vi "Mars3D_old.vi"(7 "Statemachine Data IN":T2={"Impulse Positions"=[], "Old Impulse positions for Undo"=[], "No. Imp"=0, "Parameter Time Series"=[], "Parameter Impuls Series"=[], "Experiment Parameters"={"Freq"=0.0, "Vel"=0, "Acc"=0, "Stimulus"=""}, "Autosort File"=refnum, "Data File"={"Data Channels"=[], "Sample Rate"=0, "Channel List"=[]}, "Experiment data path"=path "/Macintosh HD/Users/patrick/Studium/Diploma Thesis/Data Analysis", "Image data path"=path "/Macintosh HD/Users/patrick/Studium/Diploma Thesis/Data Analysis", "LVS data path"=path "/Macintosh HD/Users/patrick/Studium/Diploma Thesis/Data Analysis", "Raw copy path"=path "/Macintosh HD/Users/patrick/Studium/Diploma Thesis/Data Analysis", "filename"="No file selected", "desaccading parameters"={"Tolerance"=0, "Acc Range"=0.0, "Sample Rate"=0, "Impulse Plane 2"=enum."Other", "Impulse dir"=FALSE}, "Experiment Parameters 2"={"Subject"="", "Strain"="", "Rotation plane"="", "Experimenter"="", "Trial"=0.0, "Time"=0.0}, "Excel"={"Excel._Application"=refnum, "Use Excel"=FALSE, "Worksheet SINE"=refnum, "Row SINE"=0, "Worksheet TRANS"=refnum, "Row TRANS"=0}, "Session Config File"=refnum, "Autosort Parameter Set"=1, "EMA Version"="", "desacc "={"Threshold 1 [Acc]"=1617.080808080808, "Threshold 2 [% of TH1]"=67, "tolerance"=5, "Search WD "=0.19090909090909092, " always use TH2"=TRUE, "Range"=3.2323232323232323, "Max time"=200.0, "Min time"=20.0, "Velocity Threshold"=67}, "Cycle Nr for Saccades"={"POS"=0, "NEG"=0}, "Undo Counter"=0, "History Length"=0, "Redo Counter"=0, "Histpry Position"=0, "Raw Data File"={"Data Channels"=[], "Sample Rate"=0, "Channel List"=[]}, "calibration name"="No file selected"} {"Parameter Time Series"."time offset" format="%.3f"; "Parameter Time Series"."Gain" format="%.1f"; "Parameter Time Series"."Offset" format="%.1f"; "Parameter Time Series"."List 1" items=["Motor-Pos", "Motor-Vel", "Lx Position-in-Head", "Ly Position-in-Head", "Lz Position-in-Head", "Lx Velocity-in-Head", "Ly Velocity-in-Head", "Lz Velocity-in-Head", "Ll Velocity-in-Head", "Lr Velocity-in-Head", "Lx Accel-in-Head", "Ly Accel-in-Head", "Lz Accel-in-Head", "Rx Position-in-Head", "Ry Position-in-Head", "Rz Position-in-Head", "Rx Velocity-in-Head", "Ry Velocity-in-Head", "Rz Velocity-in-Head", "Rl Velocity-in-Head", "Rr Velocity-in-Head", "Rx Accel-in-Head", "Ry Accel-in-Head", "Rz Accel-in-Head", "Global Trigger", "", "", ""]; "Parameter Impuls Series"."Gain" format="%.1f"; "Parameter Impuls Series"."Offset" format="%.1f"}) -> (1 "stop 3":bool, 3 "Data Output":T1={"Data Channels"=array24x25400[609600 elements], "Sample Rate"=200, "Channel List"=["Chair Position", "Chair Velocity", "Lx Position-in-Head", "Ly Position-in-Head", "Lz Position-in-Head", "Lx Velocity-in-Head", "Ly Velocity-in-Head", "Lz Velocity-in-Head", "Ll Velocity-in-Head", "Lr Velocity-in-Head", "Lx Accel-in-Head", "Ly Accel-in-Head", "Lz Accel-in-Head", "Rx Position-in-Head", "Ry Position-in-Head", "Rz Position-in-Head", "Rx Velocity-in-Head", "Ry Velocity-in-Head", "Rz Velocity-in-Head", "Rl Velocity-in-Head", "Rr Velocity-in-Head", "Rx Accel-in-Head", "Ry Accel-in-Head", "Rz Accel-in-Head"]} {"Data Channels" format="%.2f"}, 5 "Statemachine Data OUT":T2={"Impulse Positions"=[], "Old Impulse positions for Undo"=[], "No. Imp"=0, "Parameter Time Series"=[], "Parameter Impuls Series"=[], "Experiment Parameters"={"Freq"=0.0, "Vel"=0, "Acc"=0, "Stimulus"=""}, "Autosort File"=refnum, "Data File"={"Data Channels"=[], "Sample Rate"=0, "Channel List"=[]}, "Experiment data path"=path "/Macintosh HD/Users/patrick/Studium/Diploma Thesis/Data Analysis", "Image data path"=path "/Macintosh HD/Users/patrick/Studium/Diploma Thesis/Data Analysis", "LVS data path"=path "/Macintosh HD/Users/patrick/Studium/Diploma Thesis/Data Analysis", "Raw copy path"=path "/Macintosh HD/Users/patrick/Studium/Diploma Thesis/Data Analysis", "filename"="No file selected", "desaccading parameters"={"Tolerance"=0, "Acc Range"=0.0, "Sample Rate"=0, "Impulse Plane 2"=enum."Other", "Impulse dir"=FALSE}, "Experiment Parameters 2"={"Subject"="", "Strain"="", "Rotation plane"="", "Experimenter"="", "Trial"=0.0, "Time"=0.0}, "Excel"={"Excel._Application"=refnum, "Use Excel"=FALSE, "Worksheet SINE"=refnum, "Row SINE"=0, "Worksheet TRANS"=refnum, "Row TRANS"=0}, "Session Config File"=refnum, "Autosort Parameter Set"=1, "EMA Version"="", "desacc "={"Threshold 1 [Acc]"=1617.080808080808, "Threshold 2 [% of TH1]"=67, "tolerance"=5, "Search WD "=0.19090909090909092, " always use TH2"=TRUE, "Range"=3.2323232323232323, "Max time"=200.0, "Min time"=20.0, "Velocity Threshold"=67}, "Cycle Nr for Saccades"={"POS"=0, "NEG"=0}, "Undo Counter"=0, "History Length"=0, "Redo Counter"=0, "Histpry Position"=0, "Raw Data File"={"Data Channels"=[], "Sample Rate"=0, "Channel List"=[]}, "calibration name"="No file selected"} {"Parameter Time Series"."time offset" format="%.3f"; "Parameter Time Series"."Gain" format="%.1f"; "Parameter Time Series"."Offset" format="%.1f"; "Parameter Time Series"."List 1" items=["Motor-Pos", "Motor-Vel", "Lx Position-in-Head", "Ly Position-in-Head", "Lz Position-in-Head", "Lx Velocity-in-Head", "Ly Velocity-in-Head", "Lz Velocity-in-Head", "Ll Velocity-in-Head", "Lr Velocity-in-Head", "Lx Accel-in-Head", "Ly Accel-in-Head", "Lz Accel-in-Head", "Rx Position-in-Head", "Ry Position-in-Head", "Rz Position-in-Head", "Rx Velocity-in-Head", "Ry Velocity-in-Head", "Rz Velocity-in-Head", "Rl Velocity-in-Head", "Rr Velocity-in-Head", "Rx Accel-in-Head", "Ry Accel-in-Head", "Rz Accel-in-Head", "Global Trigger", "", "", ""]; "Parameter Impuls Series"."Gain" format="%.1f"; "Parameter Impuls Series"."Offset" format="%.1f"})   [LabVIEW 2016]
uses:
  core/type-defs/TD_Statemachine-Data.ctl
  core/type-defs/TD_Time Series.ctl
  core/type-defs/TD_Impulse Parameter.ctl
  <vilib>/Utility/file.llb/Read From Spreadsheet File (DBL).vi
  tracking algorithmus/3 dot tracker.lvlib
  core/core.lvlib
panel:
  in  "stop 2":bool
  in  "VOG system":enum16{"Mouse", "Chinchilla"}(ring)
  in  "Tab Control":T5(tab)
  in  "Right Eye":T6 {"y" format="%.2f"; "z" format="%.2f"; "theta" format="%.2f"; "phi" format="%.2f"; "d" format="%.2f"}
  in  "Left Eye":T6 {"y" format="%.2f"; "z" format="%.2f"; "theta" format="%.2f"; "phi" format="%.2f"; "d" format="%.2f"}
  in  "Position Convention":u16(ring)=1 items=["Fick Angles", "Rotation Vectors"]
  in  "Angles":bool
  in  "Time Stamp":timestamp
  in  "Savgol":bool
  in  "Plot Selection":T3 {"time offset" format="%.3f"; "Gain" format="%.1f"; "Offset" format="%.1f"; "List 1" items=["Motor-Pos", "Motor-Vel", "Lx Position-in-Head", "Ly Position-in-Head", "Lz Position-in-Head", "Lx Velocity-in-Head", "Ly Velocity-in-Head", "Lz Velocity-in-Head", "Ll Velocity-in-Head", "Lr Velocity-in-Head", "Lx Accel-in-Head", "Ly Accel-in-Head", "Lz Accel-in-Head", "Rx Position-in-Head", "Ry Position-in-Head", "Rz Position-in-Head", "Rx Velocity-in-Head", "Ry Velocity-in-Head", "Rz Velocity-in-Head", "Rl Velocity-in-Head", "Rr Velocity-in-Head", "Rx Accel-in-Head", "Ry Accel-in-Head", "Rz Accel-in-Head", "Global Trigger", "", "", ""]}
  in  "Plot Selection 2":T4=[{"Color"=4652800, "Visible"=TRUE, "Channel"=1, "Invert"=FALSE, "Desaccade"=FALSE, "Offset"=0.0, "Gain"=1.0}, {"Color"=16860, "Visible"=TRUE, "Channel"=7, "Invert"=FALSE, "Desaccade"=FALSE, "Offset"=0.0, "Gain"=1.0}, {"Color"=16711680, "Visible"=TRUE, "Channel"=18, "Invert"=FALSE, "Desaccade"=FALSE, "Offset"=0.0, "Gain"=1.0}] {"Gain" format="%.1f"; "Offset" format="%.1f"}
  in  "Tolerance":i32(slide)=40 step=2 scale=0.0..100.0
  in  "Acc Range":dbl(slide)=3000.0 step=50.0 scale=0.0..30000.0
  in  "Impulse dir":bool
  in  "Impulse Plane 2":T7(ring)=enum."Yaw" caption="Impulse Plane"
  in  "process":bool
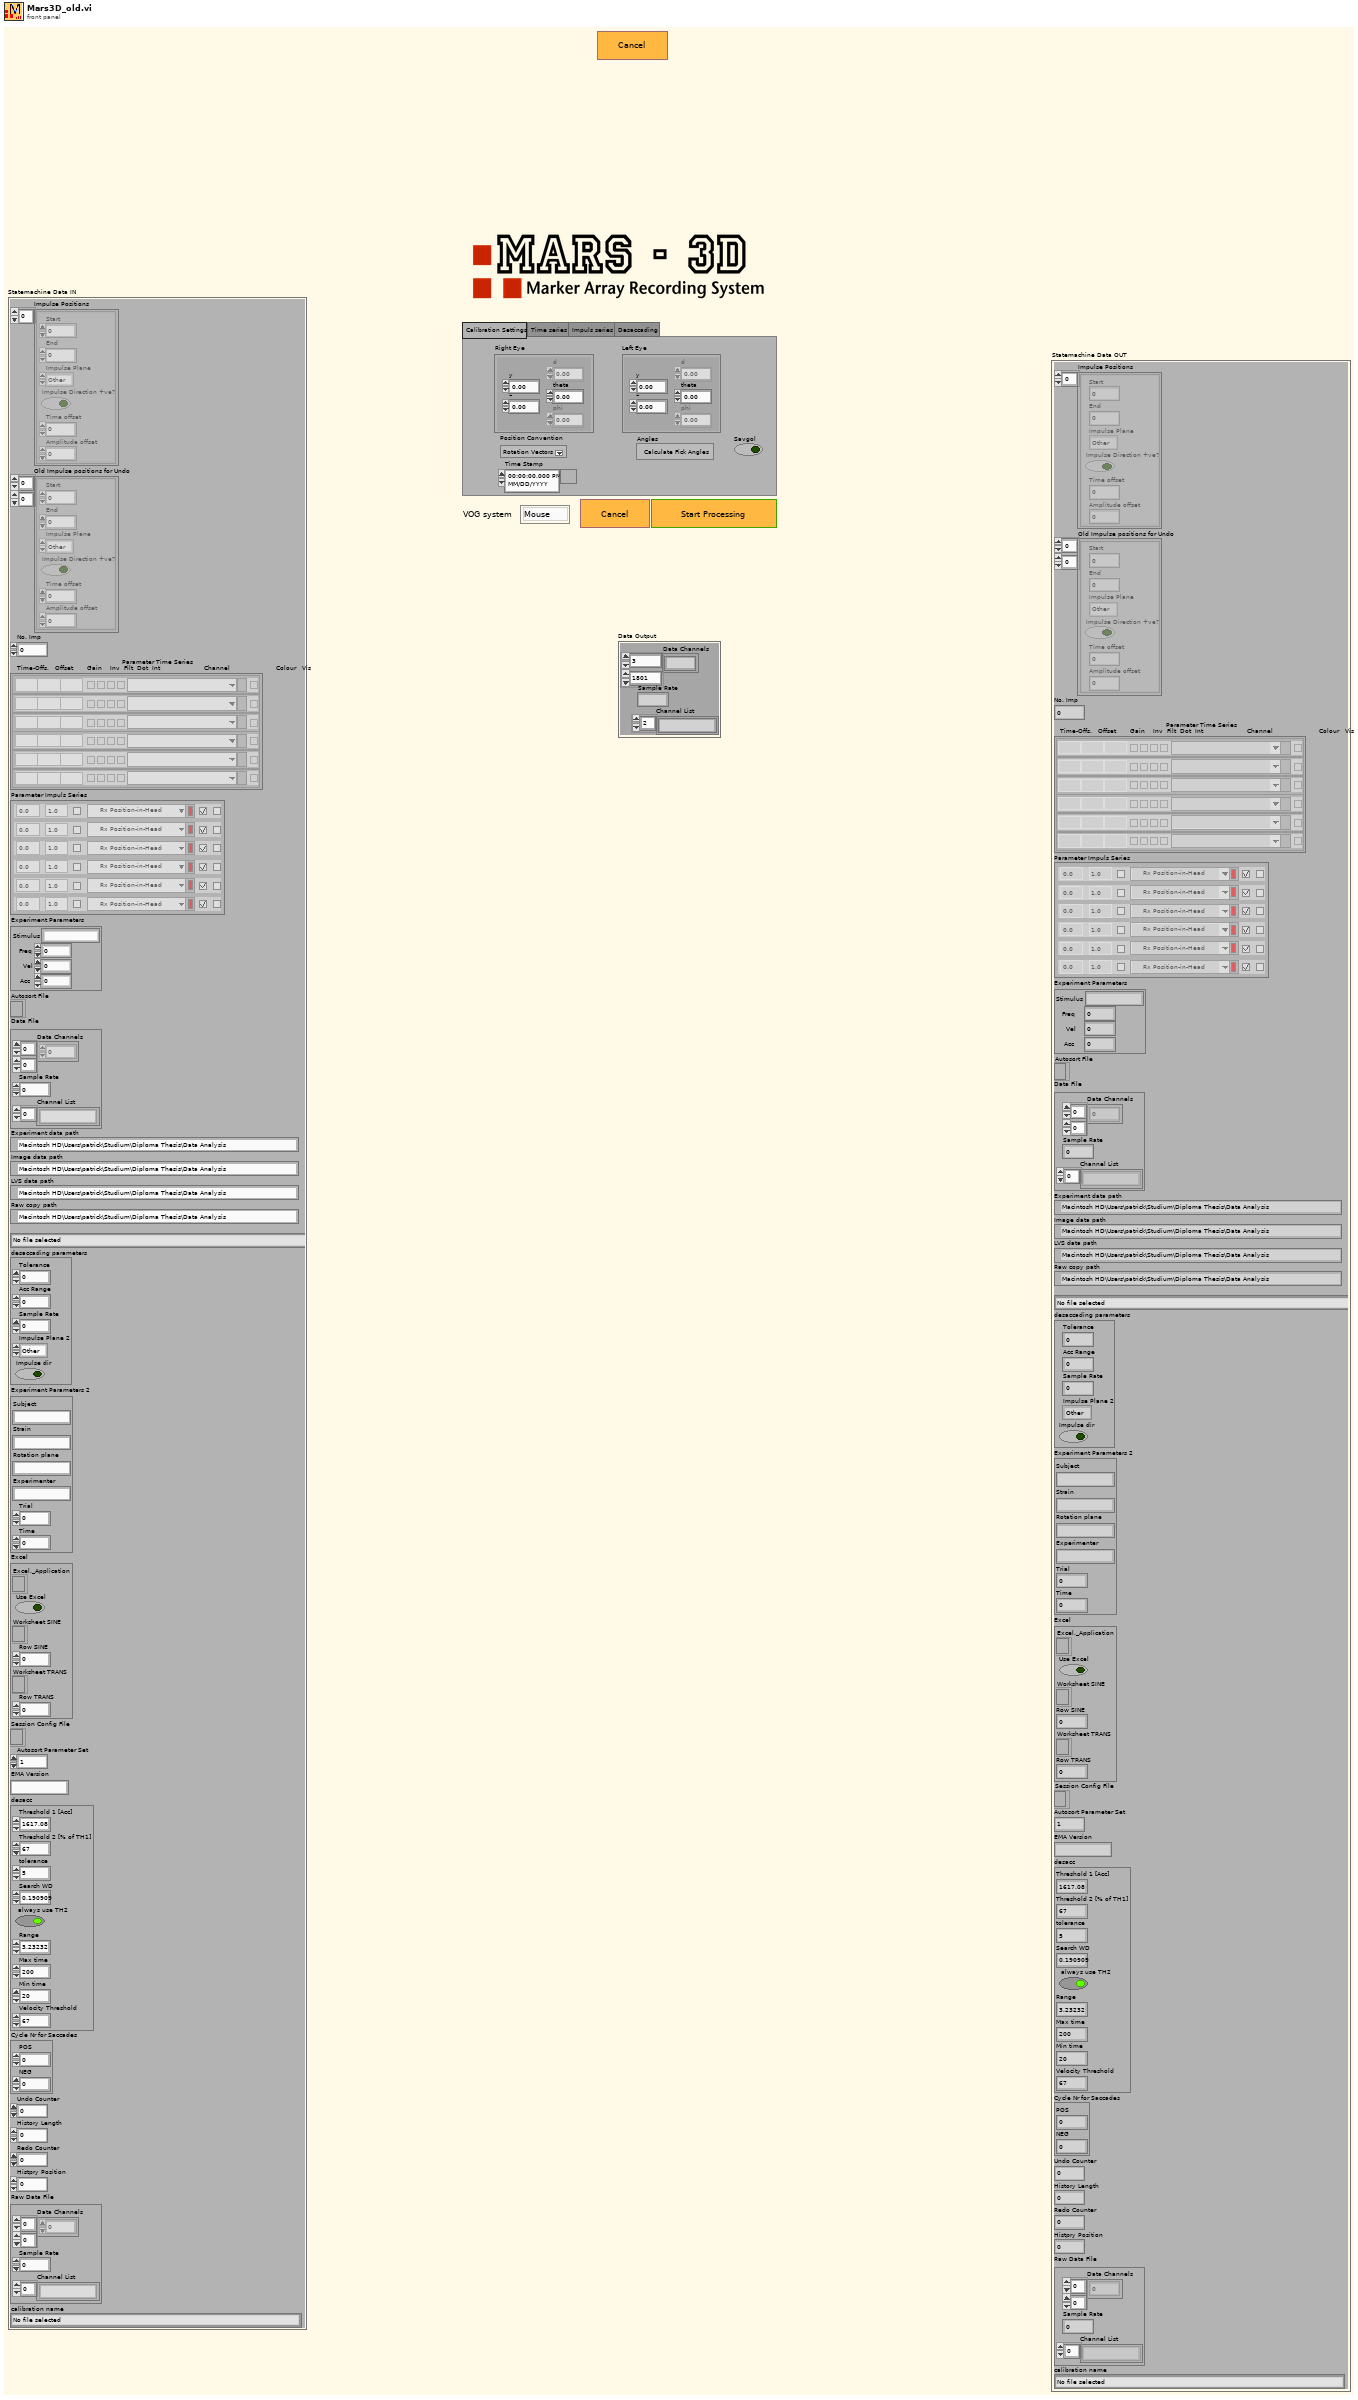
[diagram p1: front panel]
types:
  T1 = cluster{"Data Channels":dbl[][], "Sample Rate":i32, "Channel List":string[]}
  T2 = typedef "core.lvlib/TD_Statemachine-Data.ctl" = cluster{"Impulse Positions":cluster{"Start":i32, "End":i32, "Impulse Plane":enum16{"Other", "Yaw", "Pitch", "Roll", "LARP", "RALP"}, "Impulse Direction +ve?":bool, "Time offset":i32, "Amplitude offset":dbl}[], "Old Impulse positions for Undo":cluster{"Start":i32, "End":i32, "Impulse Plane":enum16{"Other", "Yaw", "Pitch", "Roll", "LARP", "RALP"}, "Impulse Direction +ve?":bool, "Time offset":i32, "Amplitude offset":dbl}[][], "No. Imp":i32, "Parameter Time Series":T3, "Parameter Impuls Series":T4, "Experiment Parameters":cluster{"Freq":dbl, "Vel":i32, "Acc":i32, "Stimulus":string}, "Autosort File":refnum<file>, "Data File":cluster{"Data Channels":dbl[][], "Sample Rate":i32, "Channel List":string[]}, "Experiment data path":path, "Image data path":path, "LVS data path":path, "Raw copy path":path, "filename":string, "desaccading parameters":cluster{"Tolerance":i32, "Acc Range":dbl, "Sample Rate":i32, "Impulse Plane 2":enum16{"Other", "Yaw", "Pitch", "Roll", "LARP", "RALP"}, "Impulse dir":bool}, "Experiment Parameters 2":cluster{"Subject":string, "Strain":string, "Rotation plane":string, "Experimenter":string, "Trial":dbl, "Time":dbl}, "Excel":cluster{"Excel._Application":refnum<k7>, "Use Excel":bool, "Worksheet SINE":refnum<k7>, "Row SINE":i32, "Worksheet TRANS":refnum<k7>, "Row TRANS":i32}, "Session Config File":refnum<file>, "Autosort Parameter Set":i32, "EMA Version":string, "desacc ":cluster{"Threshold 1 [Acc]":dbl, "Threshold 2 [% of TH1]":i32, "tolerance":i32, "Search WD ":dbl, " always use TH2":bool, "Range":dbl, "Max time":dbl, "Min time":dbl, "Velocity Threshold":i32}, "Cycle Nr for Saccades":cluster{"POS":i32, "NEG":i32}, "Undo Counter":i32, "History Length":i32, "Redo Counter":i32, "Histpry Position":i32, "Raw Data File":cluster{"Data Channels":dbl[][], "Sample Rate":i32, "Channel List":string[]}, "calibration name":string}
  T3 = typedef "core.lvlib/TD_Time Series.ctl" = cluster{"time offset":dbl, "Offset":dbl, "Gain":dbl, "inverse":bool, "filter data":bool, "dots":bool, "interpolate":bool, "List 1":u16, "Color Box":u32, "Boolean":bool}[]
  T4 = typedef "core.lvlib/TD_Impulse Parameter.ctl" = cluster{"Color":u32, "Visible":bool, "Channel":u16, "Invert":bool, "Desaccade":bool, "Offset":dbl, "Gain":dbl}[]
  T5 = enum32{"Calibration Settings", "Time series", "Impuls series", "Desaccading"}
  T6 = cluster{"d":dbl, "phi":dbl, "theta":dbl, "z":dbl, "y":dbl}
  T7 = enum16{"Other", "Yaw", "Pitch", "Roll", "LARP", "RALP"}
  T8 = cluster{"Tolerance":i32, "Acc Range":dbl, "Sample Rate":i32, "Impulse Plane 2":enum16{"Other", "Yaw", "Pitch", "Roll", "LARP", "RALP"}, "Impulse dir":bool}
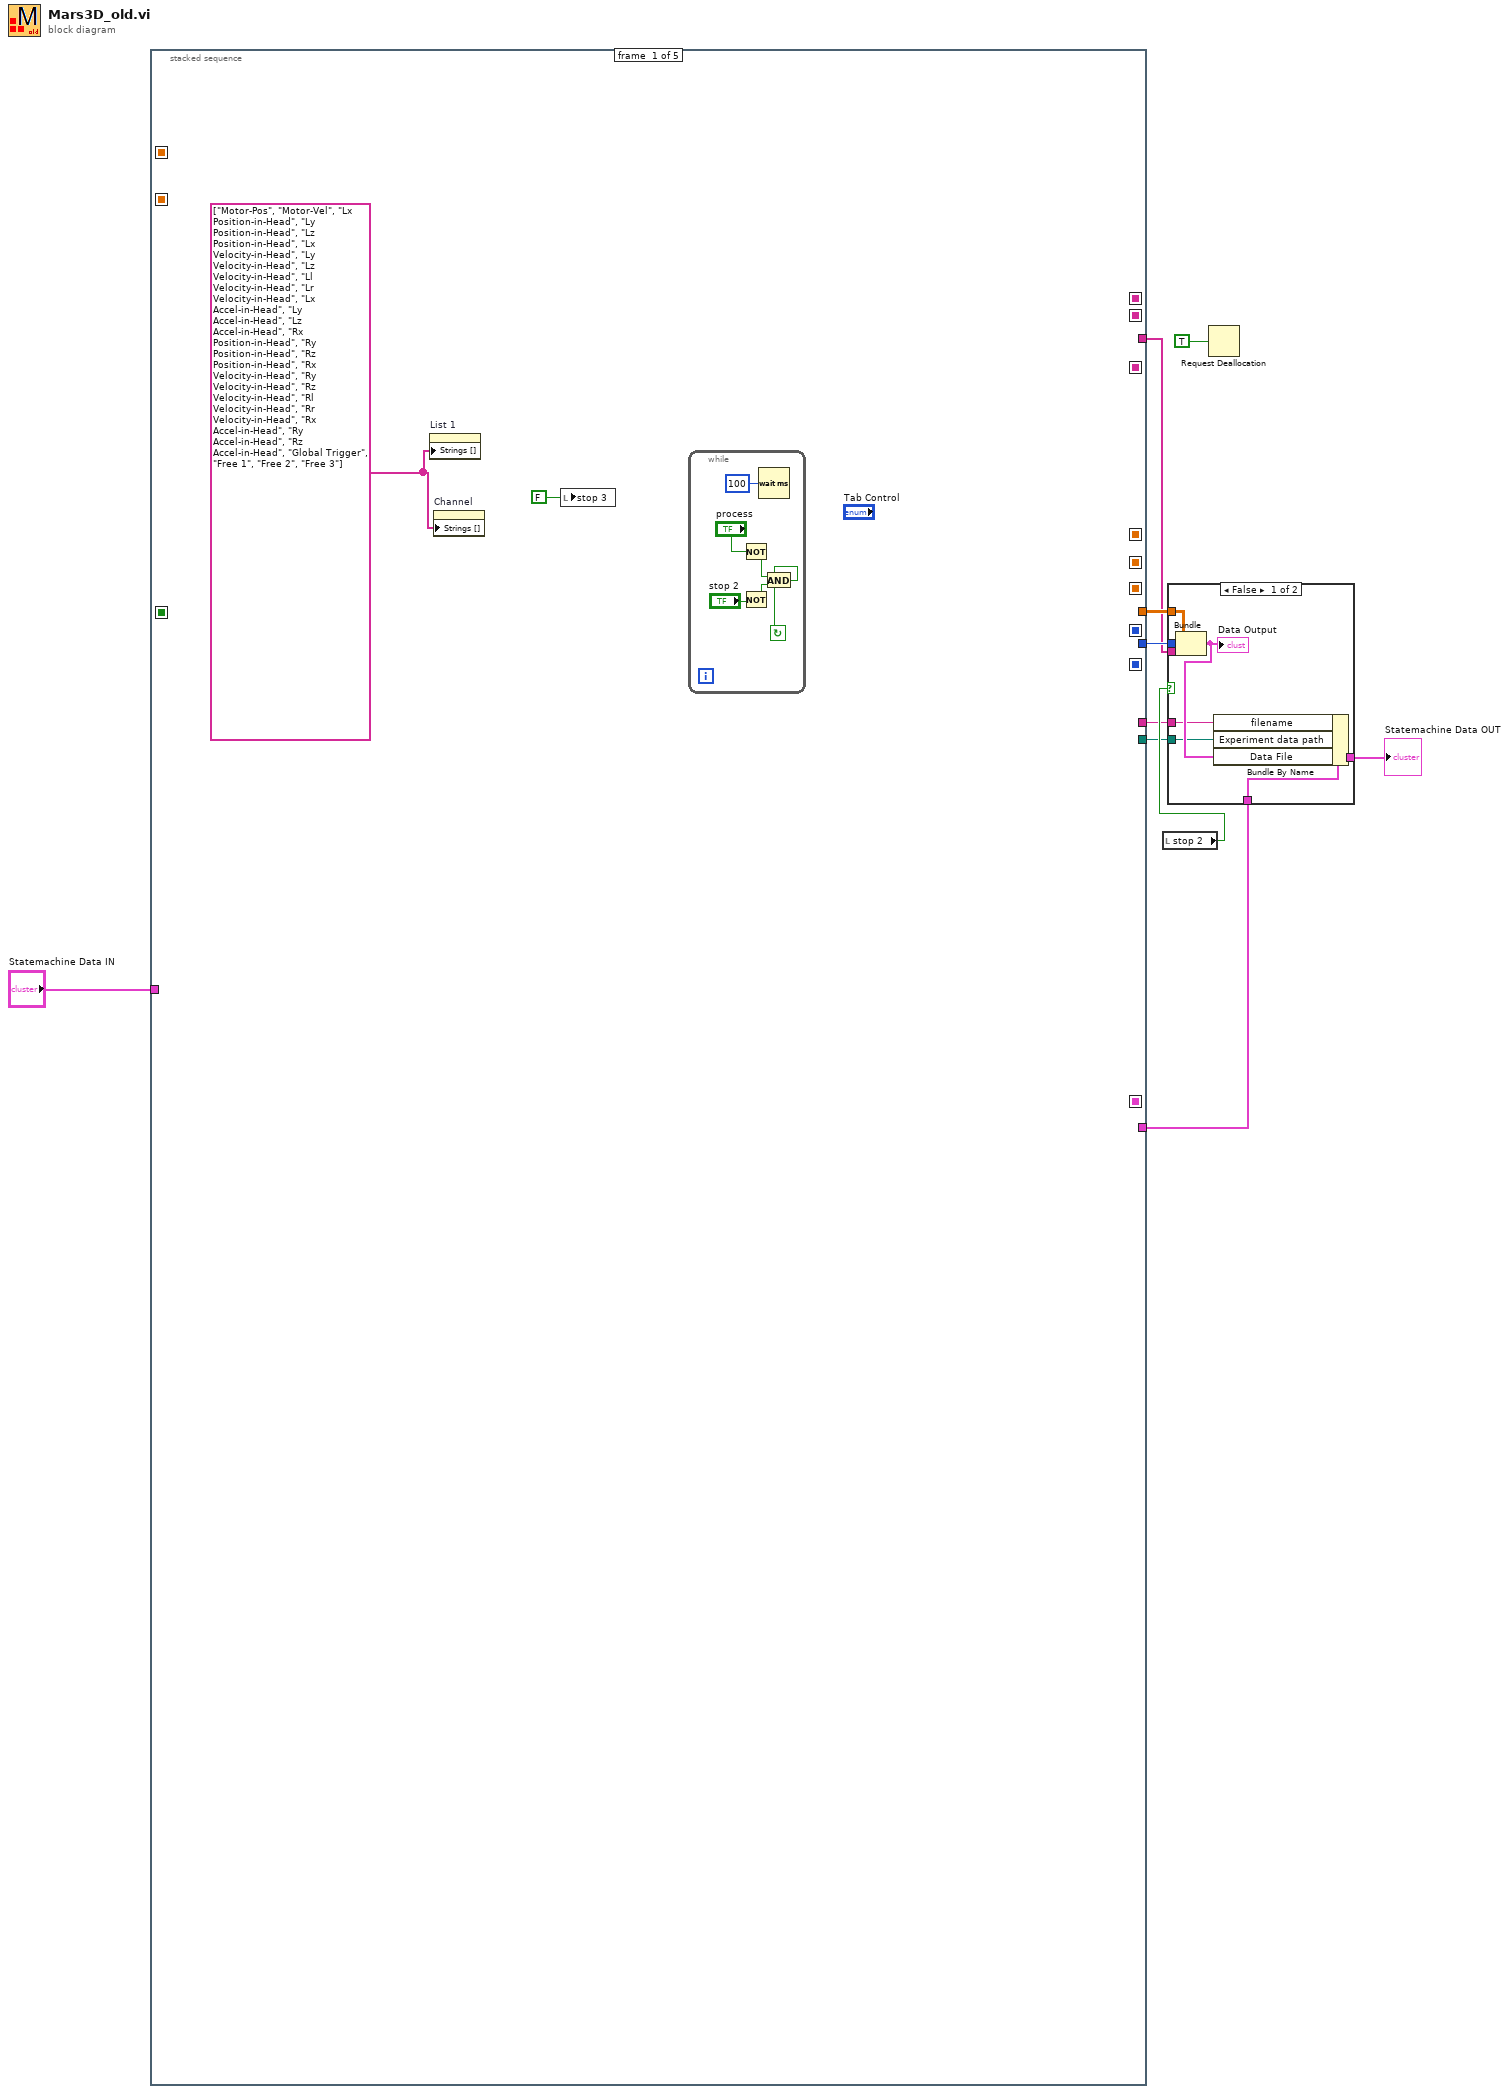
[diagram p0: block diagram]
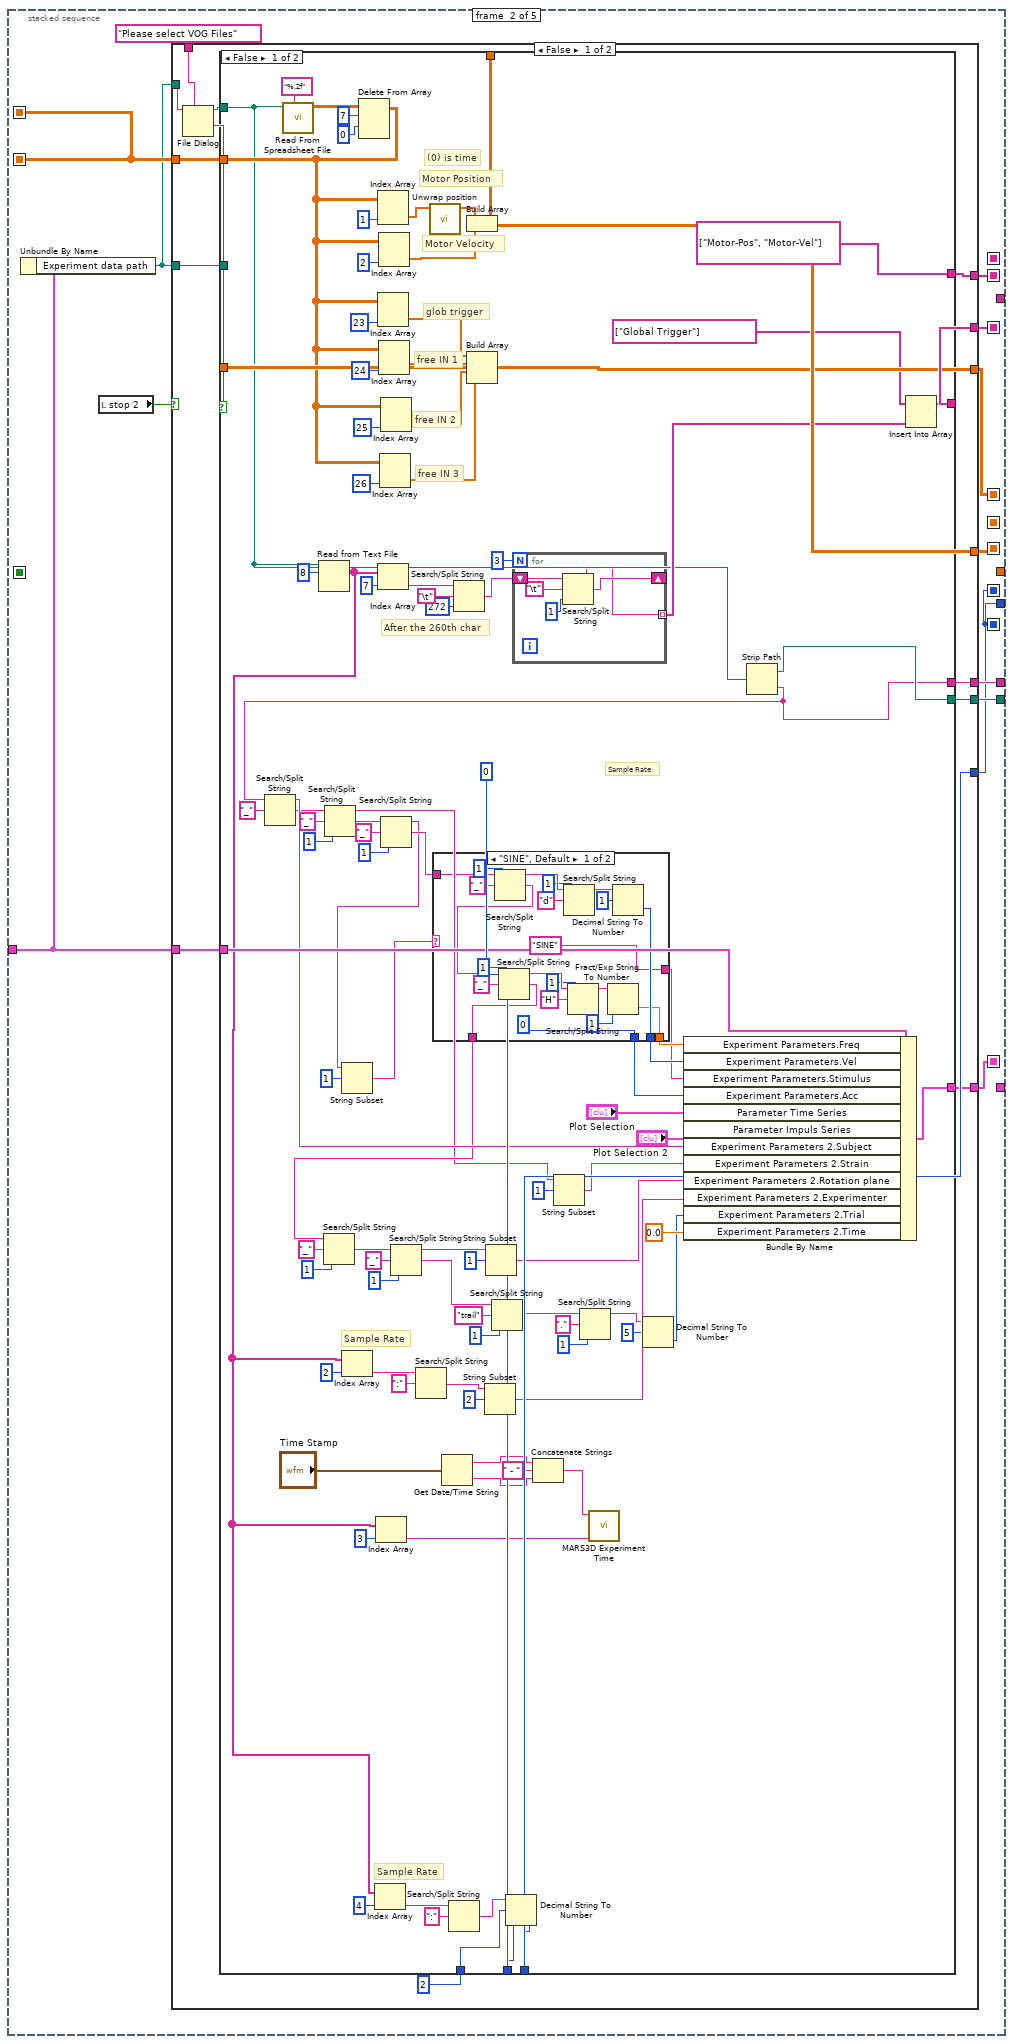
[diagram p3: hidden frame]
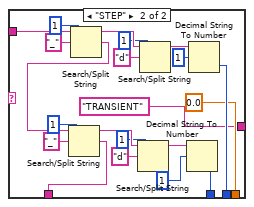
[diagram p4: hidden frame]
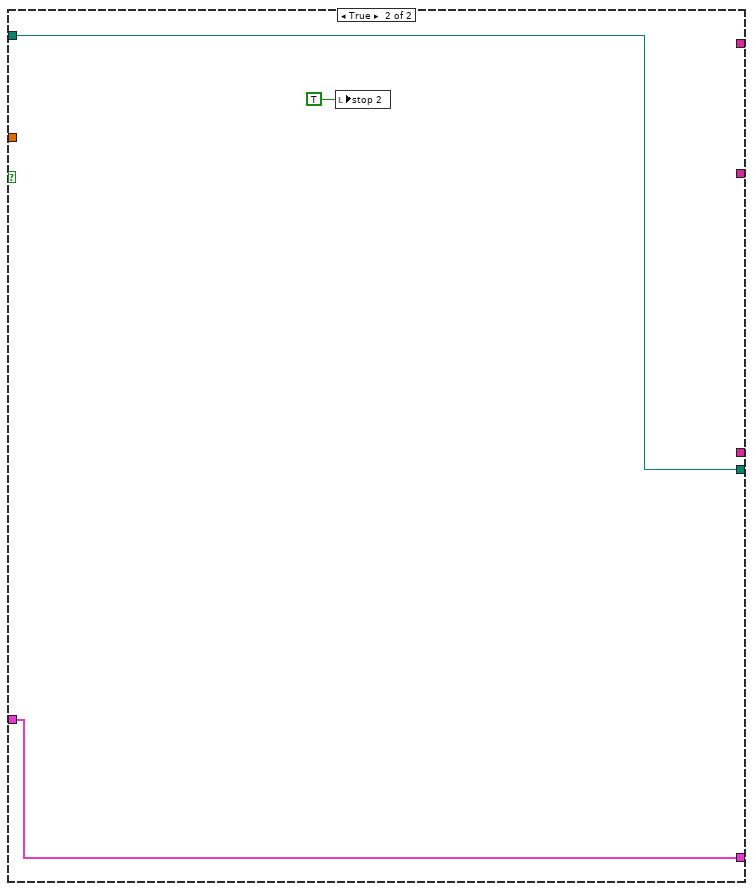
[diagram p5: hidden frame]
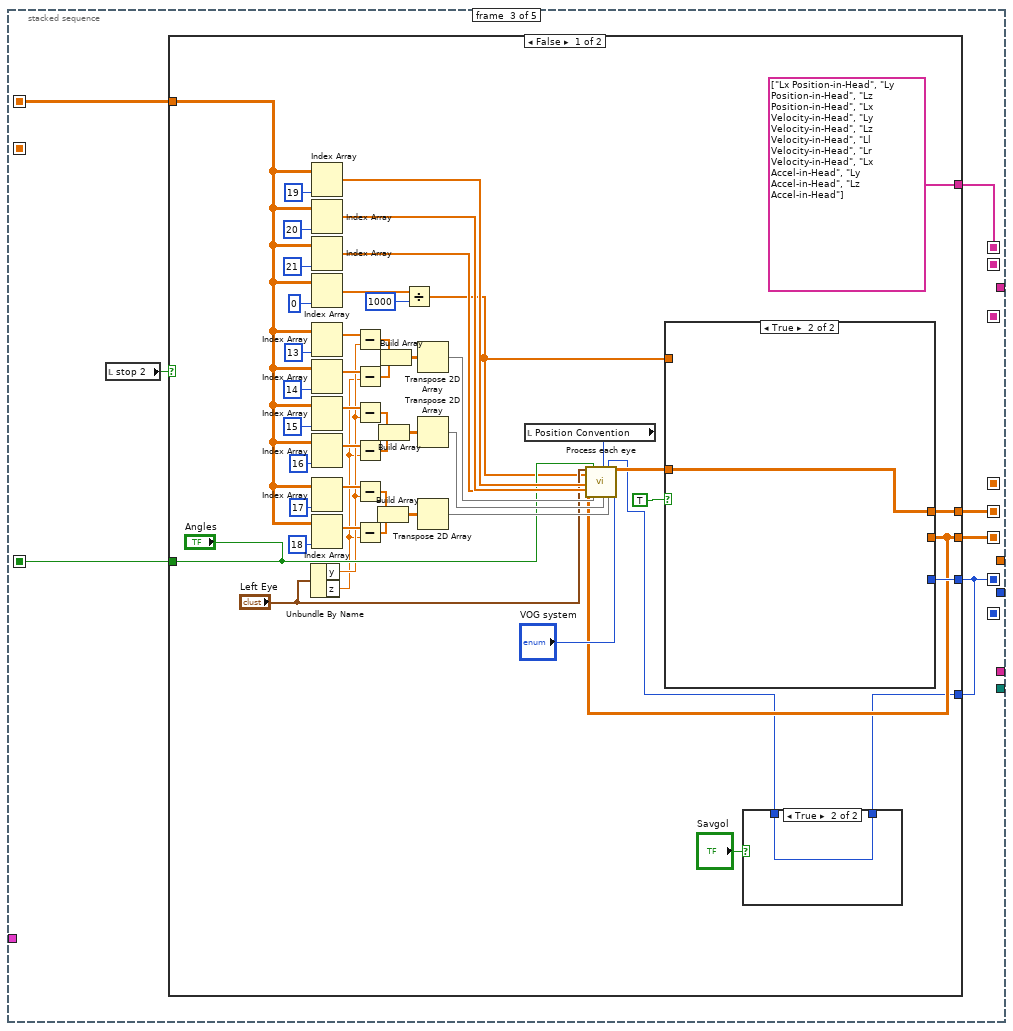
[diagram p7: hidden frame]
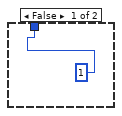
[diagram p8: hidden frame]
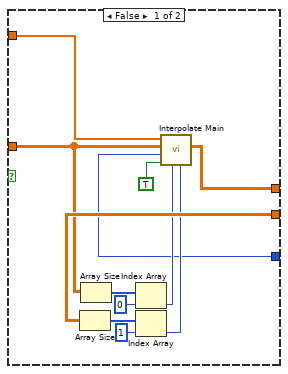
[diagram p9: hidden frame]
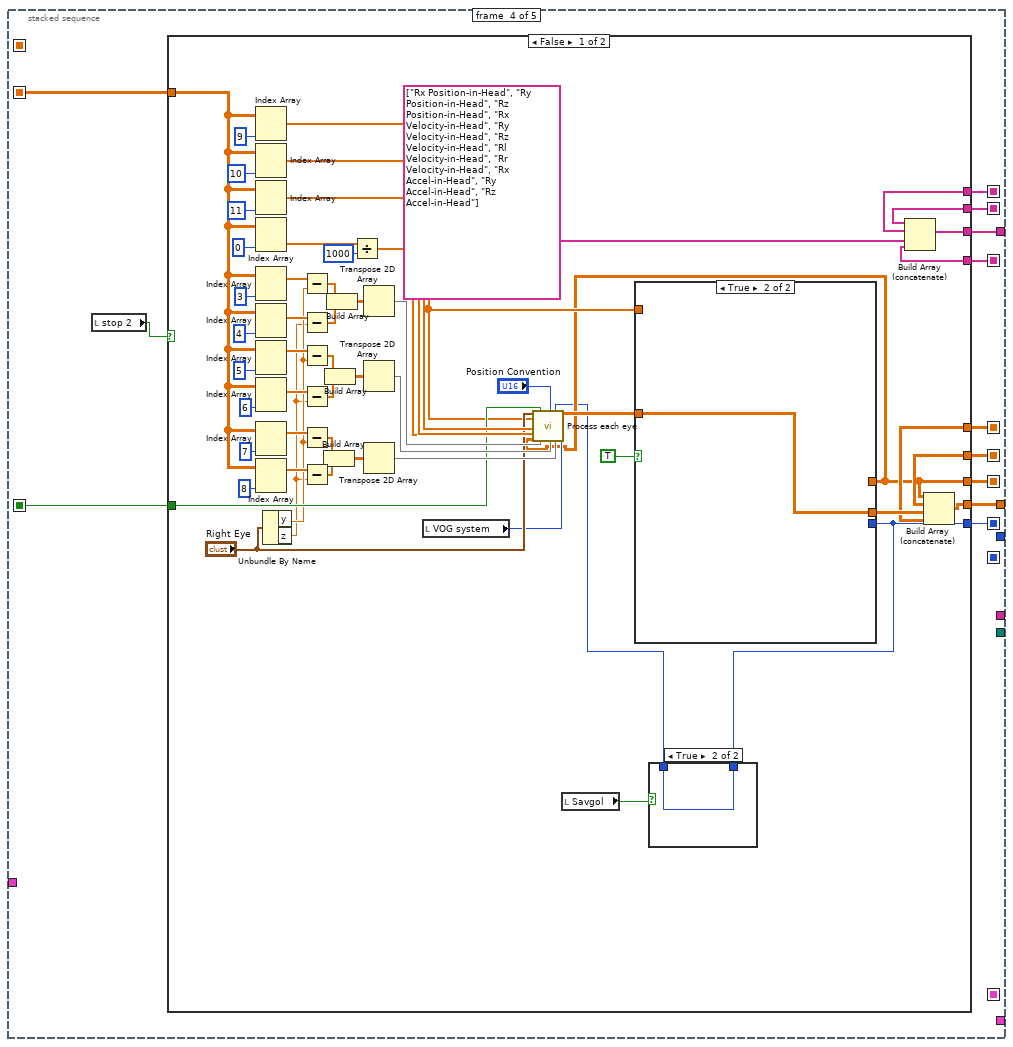
[diagram p11: hidden frame]
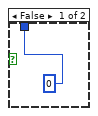
[diagram p12: hidden frame]
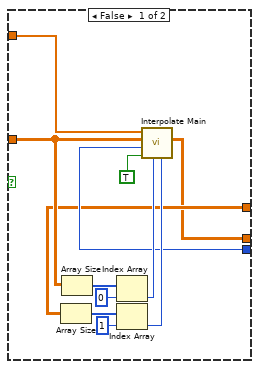
[diagram p13: hidden frame]
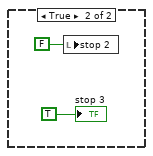
[diagram p14: hidden frame]
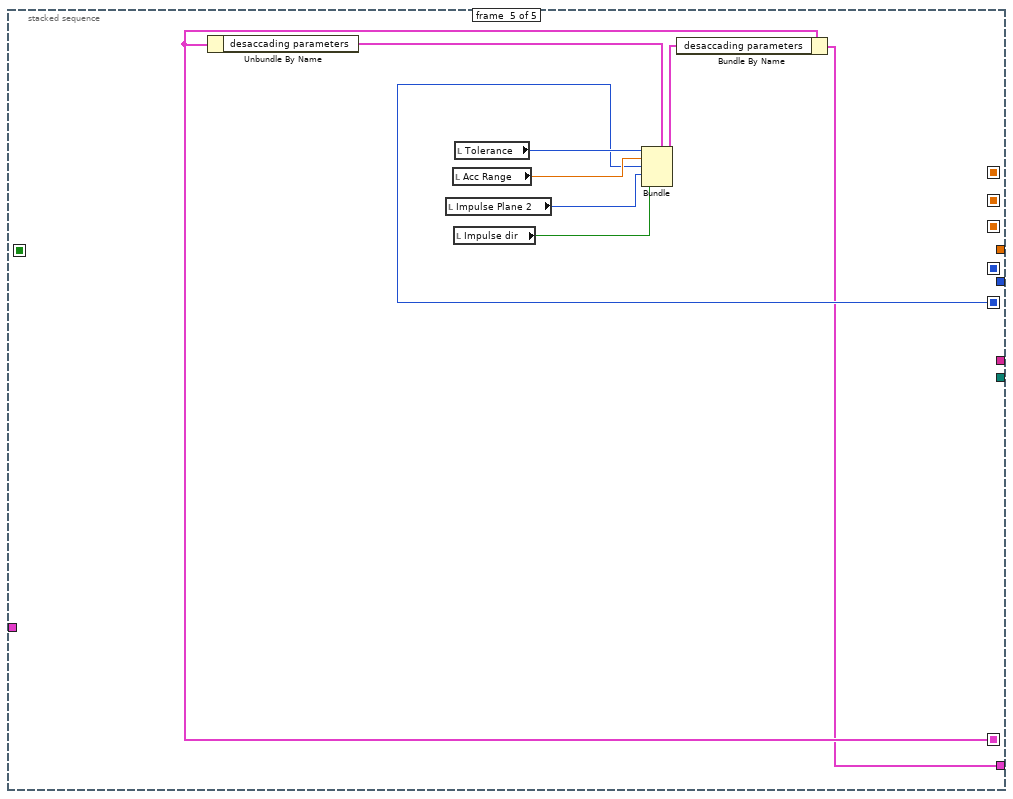
[diagram p15: hidden frame]
diagram:
  n1 = stacked-sequence {
    seq-local: [_ w31 _ _ _] -> [_ _ _ w279 _]
    seq-local: [_ w30 _ _ _] -> [_ _ w202 w274 _]
    seq-local: [_ w20 _ _ _] -> [_ _ w198 w270 _]
    seq-local: [_ w29 _ _ _] -> [_ _ _ w281 _]
    seq-local: [_ _ w204 _ _] -> [_ _ _ w280 _]
    seq-local: [_ _ w203 _ _] -> [_ _ _ w278 _]
    seq-local: [_ _ w201 _ _] -> [_ _ _ w275 _]
    seq-local: [_ w29 _ _ _] -> [_ _ w200 _ _]
    seq-local: [_ w28 _ _ _] -> [_ _ _ w272 _]
    seq-local: [_ w27 _ _ _] -> [_ _ _ w273 _]
    seq-local: [_ w20 _ _ _] -> [_ _ _ _ w360]
    seq-local: [_ w19 _ _ _] -> [_ _ _ _ w358]
    tunnel: [_ _ _ w277 _] -> w9
    tunnel: [_ _ _ w276 _] -> w7
    tunnel: [_ w20 _ _ _] -> w10
    tunnel: [_ _ _ _ w356] -> w6
    tunnel: "Statemachine Data IN" -> [_ w24 _ _ _]
    tunnel: [_ w23 _ _ _] -> w2
    tunnel: [_ w21 _ _ _] -> w1
    frame #0 {
      w11 = string[] ["Motor-Pos", "Motor-Vel", "Lx Position-in-Head", "Ly Position-in-Head", "Lz Position-in-Head", "Lx Velocity-in-Head", "Ly Velocity-in-Head", "Lz Velocity-in-Head", "Ll Velocity-in-Head", "Lr Velocity-in-Head", "Lx Accel-in-Head", "Ly Accel-in-Head", "Lz Accel-in-Head", "Rx Position-in-Head", "Ry Position-in-Head", "Rz Position-in-Head", "Rx Velocity-in-Head", "Ry Velocity-in-Head", "Rz Velocity-in-Head", "Rl Velocity-in-Head", "Rr Velocity-in-Head", "Rx Accel-in-Head", "Ry Accel-in-Head", "Rz Accel-in-Head", "Global Trigger", "Free 1", "Free 2", "Free 3"] ("Channel List")
      n2 = property on="List 1" class="Ring (strict)"("Strings []"=w11) -> ()  [unwired: 2 in, 2 out]
      n3 = property on="Channel" class="Ring (strict)"("Strings []"=w11) -> ()  [unwired: 2 in, 2 out]
      n4 = local write "stop 3"(FALSE ("stop 3")) -> ()
      n5 = while {
        stop <- w13 continue-if-true
        n6 = Not(x="process") -> (.not. x?=w14:bool)
        n7 = Not(x="stop 2") -> (.not. x?=w15:bool)
        n8 = Wait (ms)(milliseconds to wait=u32 100) -> ()  [unwired: 1 out]
        n9 = And(x=w14, y=w15) -> (x .and. y?=w13:bool)
      }
    }
    frame #1 {
      (unwired) 0 ("ADD1")
      (unwired) 0 ("ADD1")
      (unwired) 0 ("ADD1")
      n10 = Unbundle By Name(w24) -> ("Experiment data path"=w22:path)
      n11 = local read "stop 2"() -> (w26:bool)
      n12 = case shown="False" w26 {
        tunnel: [w48 _] -> w31
        tunnel: [w47 _] -> w30
        tunnel: [w45 _] -> w20
        tunnel: [w44 _] -> w29
        tunnel: [w43 _] -> w28
        tunnel: [w42 _] -> w27
        tunnel: "Please select VOG Files" ("prompt") -> [w39 _]
        tunnel: w22 -> [w37 w196]
        tunnel: [w36 w197] -> w19
        tunnel: w24 -> [w35 w197]
        tunnel: [w34 w196] -> w23
        tunnel: w22 -> [w33 _]
        tunnel: [w32 _] -> w21
        frame False {
          # "Sample Rate"
          n13 = File Dialog(7:w39, 11:w37) -> (1:w38:bool, 3:w40:path)  [unwired: 5 in, 2 out]
          n14 = case shown="False" w38 {
            tunnel: [string[] ["Motor-Pos", "Motor-Vel"] _] -> w48
            tunnel: [w139 _] -> w47
            tunnel: 0 ("default (0 I32)") -> [w133 _]
            tunnel: [w132 _] -> w45
            tunnel: [w124 _] -> w44
            tunnel: [w116 _] -> w43
            tunnel: [w110 _] -> w42
            tunnel: 2 ("offset") -> [w109 _]
            tunnel: w40 -> [w108 _]
            tunnel: [w103 w194] -> w36
            tunnel: w35 -> [w102 w194]
            tunnel: [w101 w193] -> w34
            tunnel: w33 -> [_ w193]
            tunnel: [w100 _] -> w32
            frame False {
              # "Sample Rate"
              # "Sample Rate"
              # "free IN 3"
              # "free IN 2"
              # "free IN 1"
              # "glob trigger"
              # "After the 260th char"
              # "(0) is time"
              # "Motor Velocity"
              # "Motor Position"
              n15 = call-poly <vilib>:"Read From Spreadsheet File.vi"("format (%.3f)"="%.2f", "file path (dialog if empty)"=w108) -> ("all rows"=w131:dbl[][])  [unwired: 5 in, 4 out]
              n16 = Read from Text File(file (use dialog)=w108, count=8) -> (text=w64:string[])  [unwired: 2 in, 3 out]
              n17 = Index Array(array=w64, index=2) -> (element=w75:string)
              n18 = Delete From Array(array=w131, length=7, index (row)=0) -> (array with subset deleted=w124:dbl[][])  [unwired: 1 in, 1 out]
              n19 = Index Array(array=w64, index=4) -> (element=w136:string)
              n20 = Index Array(array=w64, index=3) -> (element=w63:string)
              n21 = Index Array(array=w124, index (col)=1 ("disabled index (col)")) -> (element=w141:dbl[])  [unwired: 1 in]
              n22 = Index Array(array=w124, index (col)=23 ("disabled index (col)")) -> (element=w114:dbl[])  [unwired: 1 in]
              n23 = Index Array(array=w64, index=7) -> (element=w122:string)
              n24 = Index Array(array=w124, index (col)=2 ("disabled index (col)")) -> (element=w140:dbl[])  [unwired: 1 in]
              n25 = Index Array(array=w124, index (col)=24 ("disabled index (col)")) -> (element=w113:dbl[])  [unwired: 1 in]
              n26 = Index Array(array=w124, index (col)=26 ("disabled index (col)")) -> (element=w111:dbl[])  [unwired: 1 in]
              n27 = Index Array(array=w124, index (col)=25 ("disabled index (col)")) -> (element=w112:dbl[])  [unwired: 1 in]
              n28 = Search/Split String(string=w75, search string/char (-)=":") -> (match + rest of string=w72:string)  [unwired: 1 in, 2 out]
              n29 = call "Unwrap position.vi"("all rows"=w141) -> ("Array"=w49:sgl[])  [unwired: 10 in]
              n30 = Get Date/Time String(seconds (now)="Time Stamp") -> (date string=w61:string, time string=w59:string)  [unwired: 2 in]
              n31 = Search/Split String(string=w136, search string/char (-)=":") -> (match + rest of string=w134:string)  [unwired: 1 in, 2 out]
              n32 = Search/Split String(string=w122, search string/char (-)="\t", offset (0)=272) -> (match + rest of string=w119:string)  [unwired: 2 out]
              n33 = Build Array(w49, w140) -> (w139:dbl[][])
              n34 = Build Array(w114, w113, w112, w111) -> (w110:dbl[][])
              n35 = String Subset(string=w72, offset (0)=2) -> (substring=w71:string)  [unwired: 1 in]
              n36 = Decimal String To Number(string=w134, offset=w109, default (0L)=w133) -> (number=w132:i32)  [unwired: 1 out]
              n37 = for {
                N: 3 -> [_]
                shift-right: [w190] -> _
                shift-left: w119 -> [w192]
                tunnel: [w188] -> w115 mode=indexing
                n38 = Search/Split String(string=w192, search string/char (-)="\t", offset (0)=1) -> (substring before match=w188:string, match + rest of string=w190:string)  [unwired: 1 out]
              }
              n39 = Concatenate Strings(w61, " - " ("string"), w59) -> (w58:string)
              n40 = call "MARS3D Experiment Time.vi"("Time Experiment"=w63, "Time Calibration"=w58) -> ()  [unwired: 9 in, 1 out]
              n41 = Strip Path(path=w108) -> (stripped path=w101:path, name=w100:string)
              n42 = Search/Split String(string=w100, search string/char (-)="_") -> (substring before match=w99:string, match + rest of string=w98:string)  [unwired: 1 in, 1 out]
              n43 = Search/Split String(string=w98, search string/char (-)="_", offset (0)=1) -> (substring before match=w52:string, match + rest of string=w94:string)  [unwired: 1 out]
              n44 = Search/Split String(string=w94, search string/char (-)="_", offset (0)=1) -> (substring before match=w89:string, match + rest of string=w93:string)  [unwired: 1 out]
              n45 = String Subset(string=w89, offset (0)=1) -> (substring=w87:string)  [unwired: 1 in]
              n46 = case shown="\"SINE\", Default" w87 {
                tunnel: w93 -> [w164 w185]
                tunnel: [w160 w181] -> w92
                tunnel: [w153 0.0] -> w91
                tunnel: ["SINE" ("Experiment Parameters.Stimulus") "TRANSIENT" ("Experiment Parameters.Stimulus")] -> w86
                tunnel: [w147 w169] -> w83
                tunnel: [0 ("offset past number") w167] -> w53
                frame "SINE", Default {
                  n47 = Search/Split String(string=w164, search string/char (-)="_", offset (0)=1) -> (substring before match=w163:string, match + rest of string=w154:string)  [unwired: 1 out]
                  n48 = Search/Split String(string=w154, search string/char (-)="_", offset (0)=1) -> (substring before match=w157:string, match + rest of string=w147:string)  [unwired: 1 out]
                  n49 = Search/Split String(string=w163, search string/char (-)="d", offset (0)=1) -> (substring before match=w161:string)  [unwired: 2 out]
                  n50 = Search/Split String(string=w157, search string/char (-)="H", offset (0)=1) -> (substring before match=w159:string)  [unwired: 2 out]
                  n51 = Fract/Exp String To Number(string=w159, offset=1) -> (number=w153:dbl)  [unwired: 2 in, 1 out]
                  n52 = Decimal String To Number(string=w161, offset=1) -> (number=w160:i32)  [unwired: 1 in, 1 out]
                }
                frame "STEP" {
                  n53 = Search/Split String(string=w185, search string/char (-)="_", offset (0)=1) -> (substring before match=w184:string, match + rest of string=w175:string)  [unwired: 1 out]
                  n54 = Search/Split String(string=w175, search string/char (-)="_", offset (0)=1) -> (substring before match=w178:string, match + rest of string=w169:string)  [unwired: 1 out]
                  n55 = Search/Split String(string=w178, search string/char (-)="d", offset (0)=1) -> (substring before match=w180:string)  [unwired: 2 out]
                  n56 = Search/Split String(string=w184, search string/char (-)="d", offset (0)=1) -> (substring before match=w182:string)  [unwired: 2 out]
                  n57 = Decimal String To Number(string=w180, offset=1) -> (number=w167:i32)  [unwired: 1 in, 1 out]
                  n58 = Decimal String To Number(string=w182, offset=1) -> (number=w181:i32)  [unwired: 1 in, 1 out]
                }
              }
              n59 = Search/Split String(string=w83, search string/char (-)="_", offset (0)=1) -> (match + rest of string=w80:string)  [unwired: 2 out]
              n60 = Search/Split String(string=w80, search string/char (-)="_", offset (0)=1) -> (substring before match=w78:string, match + rest of string=w68:string)  [unwired: 1 out]
              n61 = String Subset(string=w78, offset (0)=1) -> (substring=w77:string)  [unwired: 1 in]
              n62 = Search/Split String(string=w68, search string/char (-)="trail", offset (0)=1) -> (match + rest of string=w55:string)  [unwired: 2 out]
              n63 = String Subset(string=w52, offset (0)=1) -> (substring=w51:string)  [unwired: 1 in]
              n64 = Search/Split String(string=w55, search string/char (-)=".", offset (0)=1) -> (substring before match=w54:string)  [unwired: 2 out]
              n65 = Decimal String To Number(string=w54, offset=5) -> (number=w66:i32)  [unwired: 1 in, 1 out]
              n66 = Bundle By Name(cluster=w102, "Experiment Parameters.Freq"=w91, "Experiment Parameters.Vel"=w92, "Experiment Parameters.Stimulus"=w86, "Experiment Parameters.Acc"=w53, "Parameter Time Series"="Plot Selection", "Parameter Impuls Series"="Plot Selection 2", "Experiment Parameters 2.Subject"=w99, "Experiment Parameters 2.Strain"=w51, "Experiment Parameters 2.Rotation plane"=w77, "Experiment Parameters 2.Experimenter"=w71, "Experiment Parameters 2.Trial"=w66, "Experiment Parameters 2.Time"=0.0) -> (w103:T2)
              n67 = Insert Into Array(array=string[] ["Global Trigger"], new element=w115) -> (w116:string[])  [unwired: 1 in]
            }
            frame True {
              n68 = local write "stop 2"(TRUE ("stop 2")) -> ()
            }
          }
        }
        frame True {
        }
      }
    }
    frame #2 {
      n69 = local read "stop 2"() -> (w199:bool)
      n70 = case shown="False" w199 {
        tunnel: ["Angles" _] -> w204
        tunnel: [string[] ["Lx Position-in-Head", "Ly Position-in-Head", "Lz Position-in-Head", "Lx Velocity-in-Head", "Ly Velocity-in-Head", "Lz Velocity-in-Head", "Ll Velocity-in-Head", "Lr Velocity-in-Head", "Lx Accel-in-Head", "Ly Accel-in-Head", "Lz Accel-in-Head"] _] -> w203
        tunnel: w202 -> [w208 _]
        tunnel: w198 -> [w233 _]
        tunnel: [w232 _] -> w201
        tunnel: w200 -> [w210 _]
        tunnel: w198 -> [w207 _]
        frame False {
          n71 = Unbundle By Name("Left Eye") -> ("y"=w218:dbl, "z"=w217:dbl)
          n72 = Index Array(array=w210, index (col)=19 ("index (row)")) -> (element=w243:dbl[])  [unwired: 1 in]
          n73 = Index Array(array=w210, index (col)=20 ("index (row)")) -> (element=w242:dbl[])  [unwired: 1 in]
          n74 = Index Array(array=w210, index (col)=21 ("index (row)")) -> (element=w241:dbl[])  [unwired: 1 in]
          n75 = Index Array(array=w210, index (col)=0 ("index (row)")) -> (element=w235:dbl[])  [unwired: 1 in]
          n76 = Index Array(array=w210, index (col)=13 ("index (row)")) -> (element=w230:dbl[])  [unwired: 1 in]
          n77 = Index Array(array=w210, index (col)=14 ("index (row)")) -> (element=w228:dbl[])  [unwired: 1 in]
          n78 = Index Array(array=w210, index (col)=15 ("index (row)")) -> (element=w226:dbl[])  [unwired: 1 in]
          n79 = Index Array(array=w210, index (col)=16 ("index (row)")) -> (element=w224:dbl[])  [unwired: 1 in]
          n80 = Index Array(array=w210, index (col)=17 ("index (row)")) -> (element=w222:dbl[])  [unwired: 1 in]
          n81 = Index Array(array=w210, index (col)=18 ("index (row)")) -> (element=w220:dbl[])  [unwired: 1 in]
          n82 = Subtract(x=w230, y=w218) -> (x-y=w231:dbl[])
          n83 = Subtract(x=w228, y=w217) -> (x-y=w229:dbl[])
          n84 = Subtract(x=w226, y=w218) -> (x-y=w227:dbl[])
          n85 = Subtract(x=w224, y=w217) -> (x-y=w225:dbl[])
          n86 = Subtract(x=w222, y=w218) -> (x-y=w223:dbl[])
          n87 = Subtract(x=w220, y=w217) -> (x-y=w221:dbl[])
          n88 = Build Array(w223, w221) -> (w254:dbl[][])
          n89 = Build Array(w227, w225) -> (w215:dbl[][])
          n90 = Build Array(w231, w229) -> (w216:dbl[][])
          n91 = Divide(x=w235, y=1000) -> (x/y=w212:dbl[])
          n92 = Transpose 2D Array(2D array=w216) -> (transposed array=w240:dbl[][])
          n93 = Transpose 2D Array(2D array=w215) -> (transposed array=w239:dbl[][])
          n94 = Transpose 2D Array(2D array=w254) -> (transposed array=w238:dbl[][])
          n95 = local read "Position Convention"() -> (w214:u16)
          n96 = case shown="True" "Savgol" {
            tunnel: w207 -> [_ w256]
            tunnel: [1 w256] -> w206
            frame False {
            }
            frame True {
            }
          }
          n97 = call "Process each eye.vi"("Camera coordinates rel to head co-ordinates"="Left Eye", "Time (sec)"=w212, "Hor (F)"=w243, "Ver (F)"=w242, "Posn, Vel, Acc 2"=w208, "Angles"="Angles", "Point1"=w240, "Tor (F)"=w241, "Position Convention"=w214, "Point2"=w239, "Sample Rate"=w206, "Point3"=w238, "VOG system"="VOG system") -> ("Posn, Vel, Acc"=w234:dbl[][])  [unwired: 5 in, 1 out]
          n98 = case shown="True" TRUE ("Boolean") {
            tunnel: w208 -> [w264 _]
            tunnel: w212 -> [w263 _]
            tunnel: w234 -> [w262 w269]
            tunnel: w233 -> [w259 _]
            tunnel: [w257 w269] -> w232
            frame False {
              n99 = Array Size(array=w264) -> (size(s)=w268:i32[])
              n100 = Array Size(array=w262) -> (size(s)=w267:i32[])
              n101 = Index Array(array=w267, index=0) -> (element=w261:i32)
              n102 = Index Array(array=w268, index=1) -> (element=w260:i32)
              n103 = call "Interpolate Main.vi"("Length"=w260, "Data Channels"=w261, "NaN"=TRUE, "Sample Rate"=w259, "Data"=w262, "Time"=w263) -> ("Interp Data"=w257:dbl[][])  [unwired: 4 in]
            }
            frame True {
            }
          }
        }
        frame True {
        }
      }
    }
    frame #3 {
      n104 = local read "stop 2"() -> (w271:bool)
      n105 = case shown="False" w271 {
        tunnel: w281 -> [w318 _]
        tunnel: w280 -> [w317 _]
        tunnel: w279 -> [w316 _]
        tunnel: w278 -> [w315 _]
        tunnel: [w313 _] -> w277
        tunnel: [w312 _] -> w276
        tunnel: w275 -> [w311 _]
        tunnel: w270 -> [w283 _]
        tunnel: w274 -> [w285 _]
        tunnel: w273 -> [w287 _]
        tunnel: w272 -> [w286 _]
        frame False {
          n106 = Index Array(array=w318, index (col)=9 ("index (row)")) -> (element=w324:dbl[])  [unwired: 1 in]
          n107 = Index Array(array=w318, index (col)=10 ("index (row)")) -> (element=w323:dbl[])  [unwired: 1 in]
          n108 = Index Array(array=w318, index (col)=11 ("index (row)")) -> (element=w322:dbl[])  [unwired: 1 in]
          n109 = Index Array(array=w318, index (col)=0 ("index (row)")) -> (element=w290:dbl[])  [unwired: 1 in]
          n110 = Index Array(array=w318, index (col)=3 ("index (row)")) -> (element=w300:dbl[])  [unwired: 1 in]
          n111 = Index Array(array=w318, index (col)=4 ("index (row)")) -> (element=w301:dbl[])  [unwired: 1 in]
          n112 = Index Array(array=w318, index (col)=5 ("index (row)")) -> (element=w299:dbl[])  [unwired: 1 in]
          n113 = Index Array(array=w318, index (col)=6 ("index (row)")) -> (element=w298:dbl[])  [unwired: 1 in]
          n114 = Index Array(array=w318, index (col)=7 ("index (row)")) -> (element=w297:dbl[])  [unwired: 1 in]
          n115 = Index Array(array=w318, index (col)=8 ("index (row)")) -> (element=w296:dbl[])  [unwired: 1 in]
          n116 = Unbundle By Name("Right Eye") -> ("y"=w295:dbl, "z"=w294:dbl)
          n117 = Subtract(x=w300, y=w295) -> (x-y=w307:dbl[])
          n118 = Subtract(x=w301, y=w294) -> (x-y=w306:dbl[])
          n119 = Subtract(x=w299, y=w295) -> (x-y=w305:dbl[])
          n120 = Subtract(x=w298, y=w294) -> (x-y=w304:dbl[])
          n121 = Subtract(x=w297, y=w295) -> (x-y=w303:dbl[])
          n122 = Subtract(x=w296, y=w294) -> (x-y=w302:dbl[])
          n123 = Build Array(w303, w302) -> (w337:dbl[][])
          n124 = Build Array(w305, w304) -> (w336:dbl[][])
          n125 = Build Array(w307, w306) -> (w335:dbl[][])
          n126 = Divide(x=w290, y=1000) -> (x/y=w291:dbl[])
          n127 = Transpose 2D Array(2D array=w335) -> (transposed array=w321:dbl[][])
          n128 = Transpose 2D Array(2D array=w336) -> (transposed array=w320:dbl[][])
          n129 = Transpose 2D Array(2D array=w337) -> (transposed array=w319:dbl[][])
          n130 = local read "VOG system"() -> (w292:enum16{"Mouse", "Chinchilla"})
          n131 = local read "Savgol"() -> (w282:bool)
          n132 = case shown="True" w282 {
            tunnel: [0 w339] -> w284
            tunnel: w283 -> [_ w339]
            frame False {
            }
            frame True {
            }
          }
          n133 = call "Process each eye.vi"("Camera coordinates rel to head co-ordinates"="Right Eye", "Time (sec)"=w291, "Hor (F)"=w324, "Ver (F)"=w323, "Posn, Vel, Acc 2"=w285, "Angles"=w317, "Point1"=w321, "Tor (F)"=w322, "Position Convention"="Position Convention", "Point2"=w320, "Sample Rate"=w284, "Point3"=w319, "VOG system"=w292) -> ("Posn, Vel, Acc"=w310:dbl[][])  [unwired: 5 in, 1 out]
          n134 = case shown="True" TRUE {
            tunnel: w291 -> [w344 _]
            tunnel: w310 -> [w343 w352]
            tunnel: w283 -> [w342 _]
            tunnel: w285 -> [w341 _]
            tunnel: [w340 w352] -> w309
            frame False {
              n135 = Array Size(array=w341) -> (size(s)=w351:i32[])
              n136 = Array Size(array=w343) -> (size(s)=w350:i32[])
              n137 = Index Array(array=w350, index=0) -> (element=w347:i32)
              n138 = Index Array(array=w351, index=1) -> (element=w346:i32)
              n139 = call "Interpolate Main.vi"("Length"=w346, "Data Channels"=w347, "NaN"=TRUE, "Sample Rate"=w342, "Data"=w343, "Time"=w344) -> ("Interp Data"=w340:dbl[][])  [unwired: 4 in]
            }
            frame True {
            }
          }
          n140 = Build Array (concatenate)(w316, w315, string[] ["Rx Position-in-Head", "Ry Position-in-Head", "Rz Position-in-Head", "Rx Velocity-in-Head", "Ry Velocity-in-Head", "Rz Velocity-in-Head", "Rl Velocity-in-Head", "Rr Velocity-in-Head", "Rx Accel-in-Head", "Ry Accel-in-Head", "Rz Accel-in-Head"], w286) -> (w312:string[])
          n141 = Build Array (concatenate)(w285, w311, w309, w287) -> (w313:dbl[][])
        }
        frame True {
          n142 = local write "stop 2"(FALSE ("stop 2")) -> ()
          "stop 3" <- TRUE ("stop 3")
        }
      }
    }
    frame #4 {
      n143 = Unbundle By Name(w358) -> ("desaccading parameters"=w359:T8)
      n144 = local read "Impulse Plane 2"() -> (w355:T7)
      n145 = local read "Acc Range"() -> (w362:dbl)
      n146 = local read "Impulse dir"() -> (w361:bool)
      n147 = local read "Tolerance"() -> (w363:i32)
      n148 = Bundle(cluster=w359, "Tolerance"=w363, "Acc Range"=w362, "Sample Rate"=w360, "Impulse Plane 2"=w355, "Impulse dir"=w361) -> (w357:T8)
      n149 = Bundle By Name(cluster=w358, "desaccading parameters"=w357) -> (w356:T2)
    }
  }
  n150 = local read "stop 2"() -> (w3:bool)
  n151 = case shown="False" w3 {
    tunnel: w10 -> [w371 _]
    tunnel: w9 -> [w370 _]
    tunnel: w7 -> [w369 _]
    tunnel: w6 -> [w368 w372]
    tunnel: [w367 w372] -> w5
    tunnel: w2 -> [w365 _]
    tunnel: w1 -> [w364 _]
    frame False {
      n152 = Bundle(w370, w371, w369) -> (w366:cluster{dbl[][], i32, string[]})  [unwired: 1 in]
      "Data Output" <- w366
      n153 = Bundle By Name(cluster=w368, "filename"=w364, "Experiment data path"=w365, "Data File"=w366) -> (w367:T2)
    }
    frame True {
    }
  }
  "Statemachine Data OUT" <- w5
  n154 = Request Deallocation(TRUE ("flag")) -> ()
